vi "Clear Status.vi"(0 "VISA resource name":refnum<visa-resource-name>, 11 "error in (no error)":errorcluster) -> (4 "VISA resource name out":refnum<visa-resource-name>, 15 "error out":errorcluster)   [LabVIEW 2018, in "LTB-1.lvlib" / "3150.lvlib"]
doc: "Clears the Standard Event Status Register and the Error/Event Queue."
uses:
  3150.lvlib
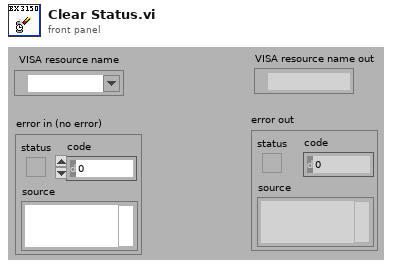
[diagram p1: front panel]
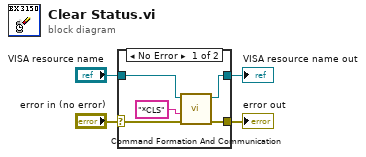
[diagram p0: block diagram]
diagram:
  n1 = case shown="No Error" "error in (no error)" {
    selector: "error in (no error)" -> [w9 w11]
    tunnel: [w8 w11] -> w1
    tunnel: [w5 w10] -> w4
    tunnel: "VISA resource name" -> [w6 w10]
    frame No Error {
      n2 = call "Command Formation And Communication.vi"("error in (no error)"=w9, "Command"="*CLS", "VISA resource name"=w6) -> ("error out"=w8:errorcluster, "VISA resource name out"=w5:refnum<visa-resource-name>)  [unwired: 1 in, 6 out]
    }
    frame Error {
    }
  }
  "VISA resource name out" <- w4
  "error out" <- w1
